vi "subGenerateFolderContainsHierarchy.vi"(10 "Path":string, 11 "Source":string) -> (1 "Label":string, 2 "New folder Id":string, 3 "Links":T1)   [LabVIEW 2020, in "DefaultExtensions.lvlib" / "CGrapherDGML.lvclass"]
uses:
  CGrapherDGML.lvclass
  obj/Addons/LabVIEWItem.lvlibp/LabVIEWItem/CLabVIEWItem/ConnectionSet.ctl
  1918f140-840c-41cb-81b1-2d34b97e3420.vi
  obj/Addons/LabVIEWItem.lvlibp/LabVIEWItem/CLabVIEWItem/CLabVIEWItem.lvclass
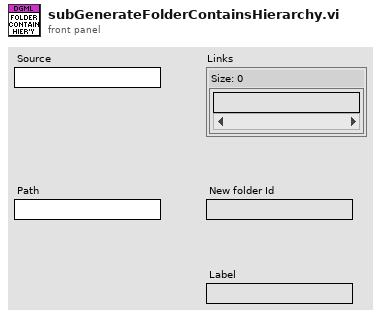
[diagram p1: front panel]
types:
  T1 = typedef "LabVIEWItem.lvlibp/CLabVIEWItem.lvclass/ConnectionSet.ctl" = set{string}
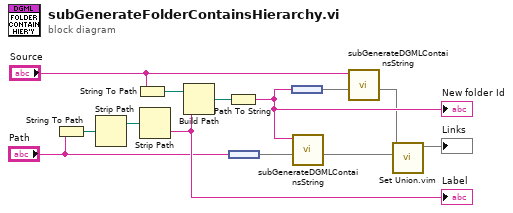
[diagram p0: block diagram]
diagram:
  n1 = String To Path(string="Path") -> (path=w12:path)
  n2 = Strip Path(path=w12) -> (stripped path=w13:path)  [unwired: 1 out]
  n3 = String To Path(string="Source") -> (path=w10:path)
  n4 = Strip Path(path=w13) -> (name=w9:string)  [unwired: 1 out]
  "Label" <- w9
  n5 = Build Path(base path=w10, name or relative path=w9) -> (appended path=w8:path)
  n6 = Path To String(path=w8) -> (string=w5:string)
  "New folder Id" <- w5
  n7 = node("Path") -> (w11:set{string})
  n8 = node(w5) -> (w4:set{string})
  n9 = call "subGenerateDGMLContainsString.vi"("Contained"=w11, "Source"=w5) -> ("Links"=w2:T1)  [unwired: 9 in]
  n10 = call "subGenerateDGMLContainsString.vi"("Contained"=w4, "Source"="Source") -> ("Links"=w3:T1)  [unwired: 9 in]
  n11 = call "Set Union.vim"("set 2"=w2, "set 1"=w3) -> ("union"=→"Links":T1)  [unwired: 9 in]
